vi "ELVIS III Check AI IRQ (FXP).vi"(5 "Hysteresis":fxp<+/-,26,5>, 6 "FIFO In":refnum<k21>="IRQ Queue", 7 "IRQ Number":u8, 8 "Threshold":fxp<+/-,26,5>, 9 "Analog Value":fxp<+/-,26,5>, 10 "Rising Edge?":bool, 11 "Enable Interrupt?":bool) -> ()   [LabVIEW 2021]
doc: "This VI checks if the analog input interrupt is triggered under the specified condition.\n<b>IRQ Number</b> specifies the identifier of the interrupt. <b>IRQ Number</b> ranges from 1 to 8 on FPGA and is shared between analog, digital, and button interrupts."
uses:
  <vilib>/Platform/TimedLoop/XDataNode/timing_clust.ctl
  <vilib>/Platform/TimedLoop/XDataNode/nitl_modes.ctl
  <vilib>/Platform/TimedLoop/XDataNode/wakeup.ctl
  <vilib>/rvi/Emulation/niFpgaSctlEmulationGetInTimedLoop.vi
  <vilib>/Utility/error.llb/Clear Errors.vi
  <vilib>/rvi/DataTransferAndStorage/Container/Common/niFpgaContainerExecOnDevCompGetState.vi
  <vilib>/rvi/Emulation/niFpgaEmulationIsFPGAContextNoSignature.vi
  <vilib>/rvi/errors/niFpgaSetErrorForExecOnDevCompSimple.vi
  <vilib>/rvi/eio/common/nirviEmuReportErrorAndStop.vi
  <vilib>/rvi/DataTransferAndStorage/Container/Common/niFpgaContainerGetUniqueNameForEmu.vi
  <vilib>/rvi/FIFO/Fifo_Resource/nirvififoEmulationSetSize.vi
  <vilib>/rvi/FIFO/Fifo_Resource/nirviFifoEmulationQueueMgr.vi
  <instcachedir>/0/nirviFifoEmulationQueueMgr_E5CAEC123FF24DC58D834DCA3CDAA9B5.lvgen/nirviFifoEmulationQueueMgr_E5CAEC123FF24DC58D834DCA3CDAA9B5_037.vi
  <vilib>/rvi/FIFO/Fifo_Resource/nirvififoEmulationDetermineInputValidOut.vi
  <vilib>/rvi/FIFO/Fifo_Resource/nirvififoEmulationCreateLock.vi
  <vilib>/rvi/Emulation/niFpgaProcessEmulError.vi
  <vilib>/rvi/FIFO/Fifo_Resource/nirvififoEmulationObtainLock.vi
  <vilib>/rvi/FIFO/Fifo_Resource/nirvififoEmulationReleaseLock.vi
  <vilib>/rvi/occurrence/nirviWaitOnOccurrenceBase.vi
  <vilib>/rvi/errors/nirviReportUnexpectedCaseInternalError.vi
  <vilib>/rvi/errors/nirviReportUnexpectedCaseInternalError (U32).vi
  <vilib>/rvi/interface/RandomDataEmulation/niFpgaRandomDataHandleErrors.vi
  <vilib>/Platform/TimedLoop/XDataNode/XDataNode.xnode
  <vilib>/rvi/DataTransferAndStorage/Container/XNode/niFpgaContainer.xnode
  <vilib>/rvi/FIFO/Fifo_Resource/niFpgaFifoEmulationRefIn.vi
  <vilib>/Platform/TimedLoop/XDataNode/XDNodeRunTimeDep.lvlib
panel:
  # "This VI checks if the analog input interrupt is triggered under the specified condition.\nIRQ Number specifies the identifier of the interrupt. IRQ Number ranges from 1 to 8 on FPGA and is shared between analog, digital, and button interrupts."
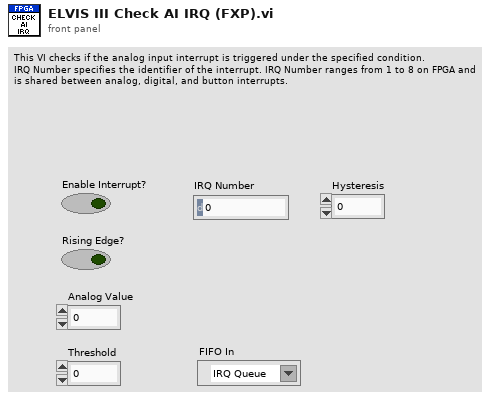
[diagram p1: front panel]
types:
  T1 = typedef "XDNodeRunTimeDep.lvlib/timing_clust.ctl" = cluster{"Expected End [f-1]":u64, "Actual End [f-1]":u64, "Finished Late? [f-1]":bool, "Expected End [i-1]":u64, "Actual End [i-1]":u64, "Finished Late? [i-1]":bool, "Expected Start [i]":u64, "Actual Start [i]":u64, "Expected Start [f]":u64, "Actual Start [f]":u64, "Source Name":string, "Structure Name":string, "Period":i64, "Deadline":i64, "Offset":i64, "Start":i64, "Priority":i32, "Timeout":i32, "Mode":T2, "Wakeup Reason":T3, "Error":errorcluster, "Source Type":string, "Secondary Source Type":string, "Global End Time":u64, "Global Start Time":u64, "Frame Duration":u64, "Iteration Duration":u64, "Assigned CPU":i32, "I/O Scan Engine Mode":u32}
  T2 = typedef "XDNodeRunTimeDep.lvlib/nitl_modes.ctl" = enum32{"No Change", "Process missed periods, maintain original phase", "Discard missed periods, maintain original phase", "Process missed periods, ignore original phase", "Discard missed periods, ignore original phase"}
  T3 = typedef "XDNodeRunTimeDep.lvlib/wakeup.ctl" = enum32{"Normal", "Aborted", "Asynchronous wakeup", "Timing source error", "Timed loop error", "Timeout"}
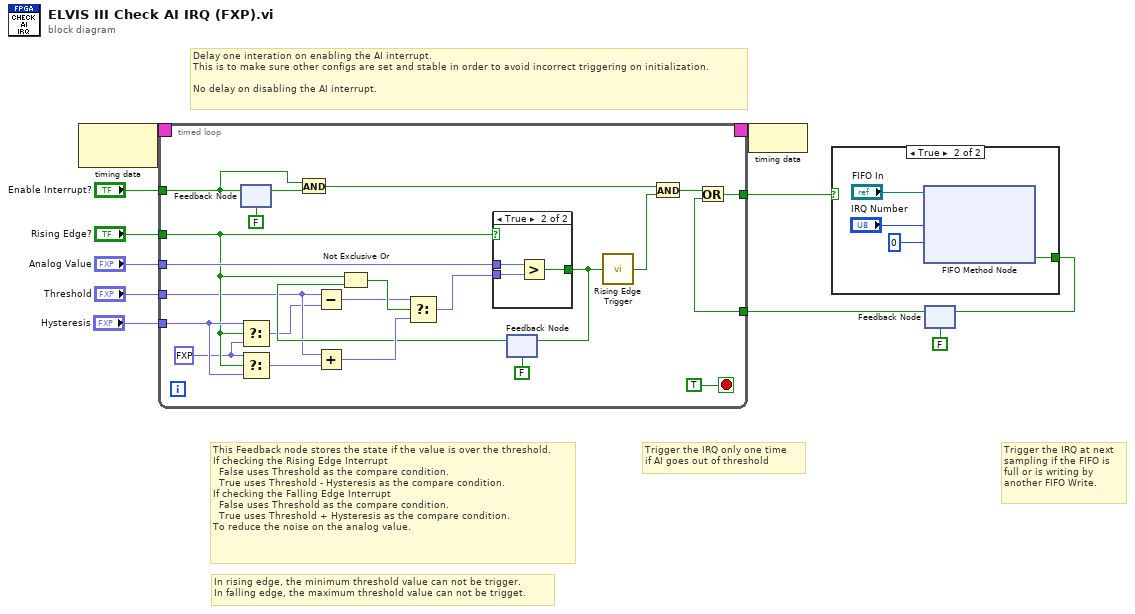
[diagram p0: block diagram]
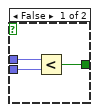
[diagram p2: hidden frame]
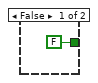
[diagram p3: hidden frame]
diagram:
  # "In rising edge, the minimum threshold value can not be trigger.\nIn falling edge, the maximum threshold value can not be trigget."
  # "Delay one interation on enabling the AI interrupt.\nThis is to make sure other configs are set and stable in order to avoid incorrect triggering on initialization.\n\nNo delay on disabling the AI interrupt."
  # "Trigger the IRQ only one time \nif AI goes out of threshold"
  # "This Feedback node stores the state if the value is over the threshold.\nIf checking the Rising Edge Interrupt\n  False uses Threshold as the compare condition.\n  True uses Threshold - Hysteresis as the compare condition.\nIf checking the Falling Edge Interrupt\n  False uses Threshold as the compare condition.\n  True uses Threshold + Hysteresis as the compare condition.\nTo reduce the noise on the analog value."
  # "Trigger the IRQ at next \nsampling if the FIFO is \nfull or is writing by \nanother FIFO Write."
  n1 = node-c288() -> (w7:T1)  [unwired: 1 in]
  n2 = feedback #1(FALSE ("Timed Out?")) -> (w2:bool)
  n3 = timed-loop {
    timing: w7 -> [_]
    timing-out: [_] -> w6
    tunnel: "Analog Value" -> [w34]
    tunnel: "Threshold" -> [w21]
    tunnel: "Hysteresis" -> [w24]
    tunnel: "Rising Edge?" -> [w23]
    tunnel: [w26] -> w3
    tunnel: w2 -> [w25]
    tunnel: "Enable Interrupt?" -> [w16]
    stop <- TRUE stop-if-true
    w19 = fxp<+/-,26,5> 0.0 ("f")
    n4 = feedback-in #2(w16) -> ()
    n5 = feedback #2(FALSE ("Enable Interrupt?")) -> (w15:bool)
    n6 = Select(t=w24, s=w23, f=w19) -> (s? t:f=w20:fxp<+/-,26,5>)
    n7 = Select(t=w19, s=w23, f=w24) -> (s? t:f=w22:fxp<+/-,26,5>)
    n8 = And(x=w16, y=w15) -> (x .and. y?=w14:bool)
    n9 = Subtract(x=w21, y=w20) -> (x-y=w12:fxp<+/-,27,6>)
    n10 = Add(x=w21, y=w22) -> (x+y=w32:fxp<+/-,27,6>)
    n11 = feedback #3(FALSE ("Timed Out?")) -> (w29:bool)
    n12 = Not Exclusive Or(1:w29, 2:w23) -> (0:w28:bool)
    n13 = Select(t=w12, s=w28, f=w32) -> (s? t:f=w31:fxp<+/-,27,6>)
    n14 = case shown="True" w23 {
      tunnel: w34 -> [w37 w40]
      tunnel: w31 -> [w36 w39]
      tunnel: [w35 w38] -> w30
      frame False {
        n15 = Less?(x=w37, y=w36) -> (x < y?=w35:bool)
      }
      frame True {
        n16 = Greater?(x=w40, y=w39) -> (0:w38:bool)
      }
    }
    n17 = feedback-in #3(w30) -> ()
    n18 = call "Rising Edge Trigger.vi"("Signal"=w30) -> ("Trigger?"=w18:bool)
    n19 = And(x=w14, y=w18) -> (x .and. y?=w17:bool)
    n20 = Or(x=w17, y=w25) -> (x .or. y?=w26:bool)
  }
  n21 = node-c288(w6) -> ()
  n22 = case shown="True" w3 {
    tunnel: [FALSE ("Timed Out?") w44] -> w5
    frame False {
    }
    frame True {
      n23 = xnode ("FIFO Method Node")("Element"="IRQ Number", "Timeout"=0, "FIFO In"="FIFO In") -> ("Timed Out?"=w44:bool)  [unwired: 1 out]
    }
  }
  n24 = feedback-in #1(w5) -> ()
